vi "slam_ortogonal_(x,y).versao3.vi"() -> ()   [LabVIEW 2016]
uses:
  <vilib>/NXT/Subs/LVHSConnector.ctl
  <vilib>/NXT/LegoClasses/BrickReference/BrickReference.lvclass
  <vilib>/NXT/Block Support/NXT_OutputPort.ctl
  <vilib>/NXT/NXTIO Xnodes/NXTIONodeSubVIs/NXTStopMotors.vi
  <vilib>/NXT/NXTIO Xnodes/NXTIONodeSubVIs/NXTMoveMotors.vi
  <vilib>/NXT/Dual Mode Library/Waits/Wait_Num.vi
  <vilib>/NXT/NXTIO Xnodes/AddressXNode/NXTIOAddress.xnode
  <vilib>/NXT/NXTIO Xnodes/NXTIOXNode/NXTIO.xnode
panel:
  out "dx":dbl format="%#_13g"
  out "dy":dbl format="%#_13g"
  out "yo":dbl format="%#_13g"
  out "xo":dbl format="%#_13g"
  out "NXT/EV3 2":T1
  in  "NXT/EV3":T1
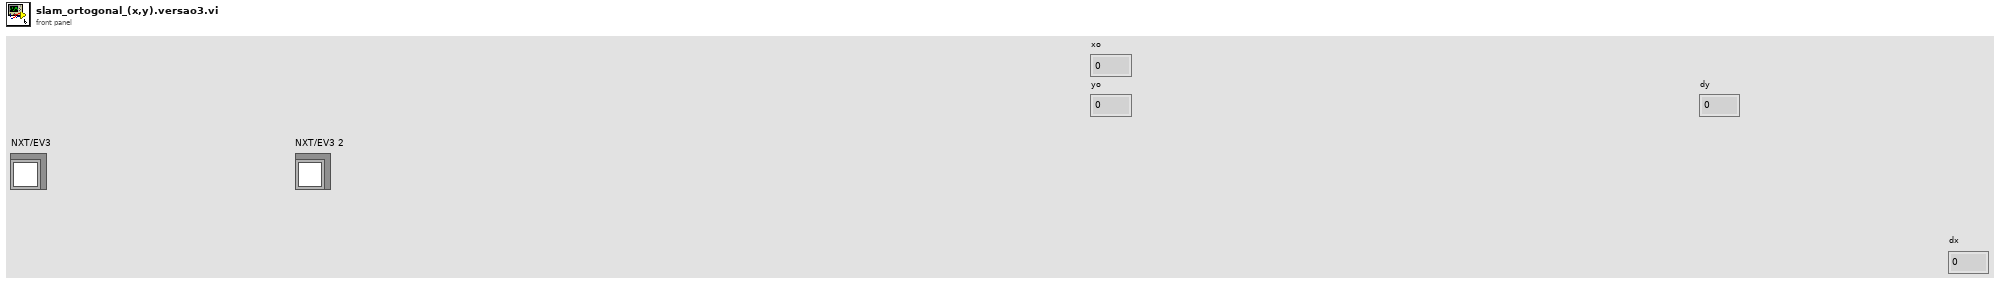
[diagram p1: front panel]
types:
  T1 = typedef "LVHSConnector.ctl" = refnum<class "BrickReference.lvclass">
  T2 = typedef "NXT_OutputPort.ctl" = u8
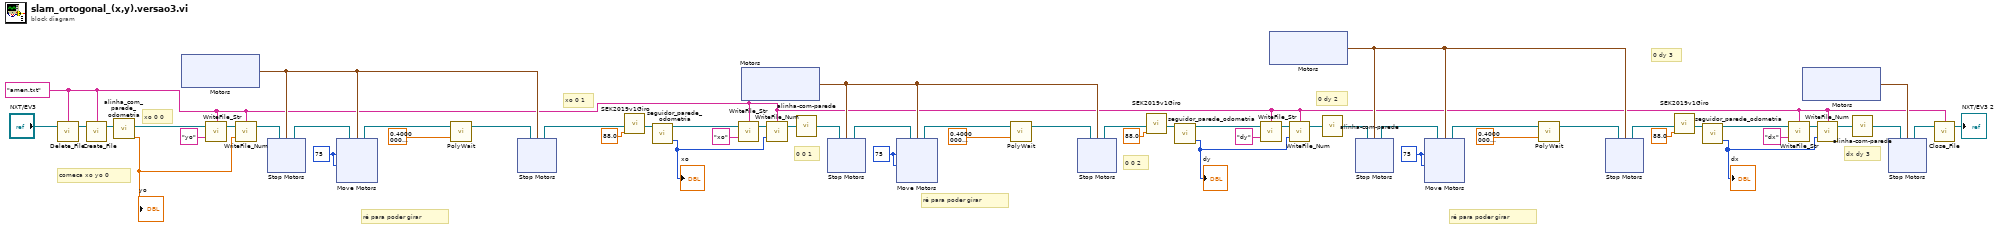
[diagram p0: block diagram]
diagram:
  w2 = "amen.txt" ("Filename")
  w34 = i8 75 ("Power/Speed 1")
  w45 = i8 75 ("Power/Speed 1")
  w53 = i8 75 ("Power/Speed 1")
  # "dx dy 3"
  # "0 dy 3"
  # "ré para poder girar"
  # "0 dy 2"
  # "0 0 2"
  # "ré para poder girar"
  # "0 0 1"
  # "xo 0 1"
  # "ré para poder girar"
  # "xo 0 0"
  # "comeca xo yo 0"
  n1 = call <vilib>:"Delete_File.vi"("NXT/EV3"="NXT/EV3", "Filename"=w2) -> ("NXT/EV3"=w26:T1)  [unwired: 2 in]
  n2 = call <vilib>:"Create_File.vi"("NXT/EV3"=w26, "Filename"=w2) -> ("NXT/EV3"=w22:T1)  [unwired: 2 in]
  n3 = call "alinha_com_parede_odometria.vi"("NXT/EV3"=w22) -> ("Numeric"=w20:dbl, "NXT/EV3 2"=w21:T1)  [unwired: 9 in]
  "yo" <- w20
  n4 = xnode "Motors"() -> ("Motor"=w49:cluster{"Port":T2, "Port":T2})
  n5 = call <vilib>:"WriteFile_Str.vi"("String"="yo", "NXT/EV3"=w21, "Filename"=w2) -> ("NXT/EV3"=w25:T1)  [unwired: 1 in]
  n6 = call <vilib>:"WriteFile_Num.vi"("Number"=w20, "NXT/EV3"=w25, "Filename"=w2) -> ("NXT/EV3"=w1:T1)  [unwired: 1 in]
  n7 = xnode "Stop Motors"("Motors"=w49, "NXT/EV3"=w1) -> ("NXT/EV3"=w54:T1)
  n8 = xnode "Move Motors"("Power/Speed 2"=w53, "Power/Speed 1"=w53, "Motors"=w49, "NXT/EV3"=w54) -> ("NXT/EV3"=w55:T1)
  n9 = call-poly <vilib>:"PolyWait.vi"("Time (1 sec)"=sgl 0.4, "NXT/EV3"=w55) -> ("NXT/EV3"=w57:T1)  [unwired: 2 in]
  n10 = xnode "Stop Motors"("Motors"=w49, "NXT/EV3"=w57) -> ("NXT/EV3"=w52:T1)
  n11 = call "SEK2019v1Giro.vi"("ANGULO"=sgl 88.0, "NXT/EV3"=w52) -> ("NXT/EV3 2"=w50:T1)  [unwired: 9 in]
  n12 = call "seguidor_parede_odometria.vi"("NXT/EV3 3"=w50) -> ("Numeric 2"=w15:i32, "NXT/EV3 2"=w19:T1)  [unwired: 3 in]
  "xo" <- w15
  n13 = call <vilib>:"WriteFile_Str.vi"("String"="xo", "NXT/EV3"=w19, "Filename"=w2) -> ("NXT/EV3"=w18:T1)  [unwired: 1 in]
  n14 = xnode "Motors"() -> ("Motor"=w48:cluster{"Port":T2, "Port":T2})
  n15 = call <vilib>:"WriteFile_Num.vi"("Number"=w15, "NXT/EV3"=w18, "Filename"=w2) -> ("NXT/EV3"=w17:T1)  [unwired: 1 in]
  n16 = call "alinha-com-parede.vi"("NXT/EV3"=w17) -> ("NXT/EV3 2"=w40:T1)  [unwired: 4 in]
  n17 = xnode "Stop Motors"("Motors"=w48, "NXT/EV3"=w40) -> ("NXT/EV3"=w44:T1)
  n18 = xnode "Move Motors"("Power/Speed 2"=w45, "Power/Speed 1"=w45, "Motors"=w48, "NXT/EV3"=w44) -> ("NXT/EV3"=w43:T1)
  n19 = call-poly <vilib>:"PolyWait.vi"("Time (1 sec)"=sgl 0.4, "NXT/EV3"=w43) -> ("NXT/EV3"=w41:T1)  [unwired: 2 in]
  n20 = xnode "Stop Motors"("Motors"=w48, "NXT/EV3"=w41) -> ("NXT/EV3"=w46:T1)
  n21 = call "SEK2019v1Giro.vi"("ANGULO"=sgl 88.0, "NXT/EV3"=w46) -> ("NXT/EV3 2"=w28:T1)  [unwired: 9 in]
  n22 = call "seguidor_parede_odometria.vi"("NXT/EV3 3"=w28) -> ("Numeric 2"=w10:i32, "NXT/EV3 2"=w13:T1)  [unwired: 3 in]
  "dy" <- w10
  n23 = call <vilib>:"WriteFile_Str.vi"("String"="dy", "NXT/EV3"=w13, "Filename"=w2) -> ("NXT/EV3"=w14:T1)  [unwired: 1 in]
  n24 = xnode "Motors"() -> ("Motor"=w29:cluster{"Port":T2, "Port":T2})
  n25 = call <vilib>:"WriteFile_Num.vi"("Number"=w10, "NXT/EV3"=w14, "Filename"=w2) -> ("NXT/EV3"=w12:T1)  [unwired: 1 in]
  n26 = call "alinha-com-parede.vi"("NXT/EV3"=w12) -> ("NXT/EV3 2"=w39:T1)  [unwired: 4 in]
  n27 = xnode "Stop Motors"("Motors"=w29, "NXT/EV3"=w39) -> ("NXT/EV3"=w35:T1)
  n28 = xnode "Move Motors"("Power/Speed 2"=w34, "Power/Speed 1"=w34, "Motors"=w29, "NXT/EV3"=w35) -> ("NXT/EV3"=w36:T1)
  n29 = call-poly <vilib>:"PolyWait.vi"("Time (1 sec)"=sgl 0.4, "NXT/EV3"=w36) -> ("NXT/EV3"=w38:T1)  [unwired: 2 in]
  n30 = xnode "Stop Motors"("Motors"=w29, "NXT/EV3"=w38) -> ("NXT/EV3"=w33:T1)
  n31 = call "SEK2019v1Giro.vi"("ANGULO"=sgl 88.0, "NXT/EV3"=w33) -> ("NXT/EV3 2"=w27:T1)  [unwired: 9 in]
  n32 = call "seguidor_parede_odometria.vi"("NXT/EV3 3"=w27) -> ("Numeric 2"=w5:i32, "NXT/EV3 2"=w7:T1)  [unwired: 3 in]
  "dx" <- w5
  n33 = call <vilib>:"WriteFile_Str.vi"("String"="dx", "NXT/EV3"=w7, "Filename"=w2) -> ("NXT/EV3"=w8:T1)  [unwired: 1 in]
  n34 = xnode "Motors"() -> ("Motor"=w31:cluster{"Port":T2, "Port":T2})
  n35 = call <vilib>:"WriteFile_Num.vi"("Number"=w5, "NXT/EV3"=w8, "Filename"=w2) -> ("NXT/EV3"=w6:T1)  [unwired: 1 in]
  n36 = call "alinha-com-parede.vi"("NXT/EV3"=w6) -> ("NXT/EV3 2"=w30:T1)  [unwired: 4 in]
  n37 = xnode "Stop Motors"("Motors"=w31, "NXT/EV3"=w30) -> ("NXT/EV3"=w4:T1)
  n38 = call <vilib>:"Close_File.vi"("NXT/EV3"=w4, "Filename"=w2) -> ("NXT/EV3"=→"NXT/EV3 2":T1)  [unwired: 2 in]
